vi "PicoScope5000aExampleRapidBlockBulkOverlapped.vi"() -> ()   [LabVIEW 2020]
uses:
  shared/Acquisition Settings.ctl
  shared/Buffer and Transfer Settings.ctl
  shared/nSegments.ctl
  shared/Segment Range.ctl
  PicoScope5000aLib/PicoScope5000aAnalogChannelSettings.ctl
  PicoScope5000aLib/PicoScope5000aDigitalChannelSettings.ctl
  shared/PicoBuffers.ctl
  <vilib>/Waveform/DWDTOps.llb/DWDT Analog to Digital.vi
panel:
  out "overflow":i16[](array[numeric]) format="%06b"
  in  "Port 0 Settings":T1={"Enabled"=FALSE, "Logic Level"=9830} {"Logic Level" items=["1.5V TTL"=9830, "2.5V CMOS"=16383]}
  in  "Channel A Settings":T2={"Enabled"=TRUE, "Coupling"=1, "Range"=6, "Analogue Offset"=0.0, "Bandwidth Limit"=0} {"Bandwidth Limit" items=["Full", "20MHz"]; "Range" items=["10 mV", "20 mV", "50 mV", "100 mV", "200 mV", "500 mV", "1 V", "2 V", "5 V", "10 V", "20 V"]; "Coupling" items=["AC", "DC"]}
  in  "Trigger Settings":T3={"Trigger Enabled"=FALSE, "Trigger Source"=enum."Channel A", "Trigger Threshold (volts)"=0.0, "Trigger Direction"=2, "Trigger Delay (samples)"=0, "Auto Trigger Time (ms)"=1000} {"Trigger Direction" items=["Rising"=2, "Falling"=3]}
  out "USB 3.0 device on non-USB 3.0 Port":bool
  out "USB Powered":bool=TRUE
  out "Device Info":T4={"Driver Version"="2.1.104.3324", "USB Version"="2.0", "Hardware"="1", "Variant"="5244A", "Batch and Serial"="CQ178/007", "Cal Date"="11Jun13", "Kernel Version"="1.0", "Digital HW Version"="1", "Analogue HW Version"="1", "MSO"=FALSE, "Number of channels"=2}
  out "Trigger Offsets":cluster{"Samples":u64, "Time (seconds)":sgl}[](array[cluster]) {"Time (seconds)" format="%#_5p"}
  in  "Stop Display":bool
  out "Capture Complete":bool
  in  "Run":bool
  in  "Display Buffer Index":i32
  in  "Segment Range":T5={"fromSegmentIndex"=0, "toSegmentIndex"=9} {"toSegmentIndex" format="%.4p"; "fromSegmentIndex" format="%.4p"}
  in  "nSegments":T6=10 format="%.4p"
  out "error out":errorcluster
  in  "Data file":path=path "PicoScope5000aExampleRapidBlock ChA Data"
  in  "Buffer and Transfer Settings":T7={"startIndex"=0, "Samples"=5000000, "Down Sample Ratio"=1, "Down-Sample Mode"=0} {"Down-Sample Mode" items=["RAW none"=2147483648, "None"=0, "Aggregate"=1, "Decimate"=2, "Average"=4]; "Down Sample Ratio" step=1; "Samples" format="%_6p"}
  in  "Acquisition Settings":T8={"preTriggerSamples"=0, "postTriggerSamples"=5000000, "timebase"=5} {"postTriggerSamples" format="%_6p"; "preTriggerSamples" format="%_6p"}
  out "Properties Panel":T9={"Sample Frequency"=41666668.0, "Sample Rate"=2.4000000209412065e-08, "Max Samples Available"=26843008, "Number of Samples"=0, "Total Capture Time (sec) "=0.0, "Max Total Capture Time Available (sec)"=0.6442322134971619} {"Max Total Capture Time Available (sec)" format="%.3p"; "Sample Frequency" format="%.6p"; "Sample Rate" format="%.3p"; "Max Samples Available" format="%_6p"; "Total Capture Time (sec)" format="%.3p"}
  out "Port 0":digitalwaveform(graph)={"t0"=timestamp(0 s since 1904-01-01), "dt"=8e-09, "Y"={"transitions"=[], "data"=[]}}
  in  "stop":bool
  out "Analog Channels":cluster{i32, sgl, "Data":dbl[]}[](graph)
  in  "Resolution":u32(ring) items=["8-bit"=0, "12-bit"=1, "14-bit"=2, "15-bit"=3, "16-bit"=4, "10-bit"=10]
  in  "Serial Number":string
  in  "Use Serial Number":bool
  in  "error in (no error)":errorcluster
  # "Number of\nSegments to Capture"
  # "Bit 0 = ChA"
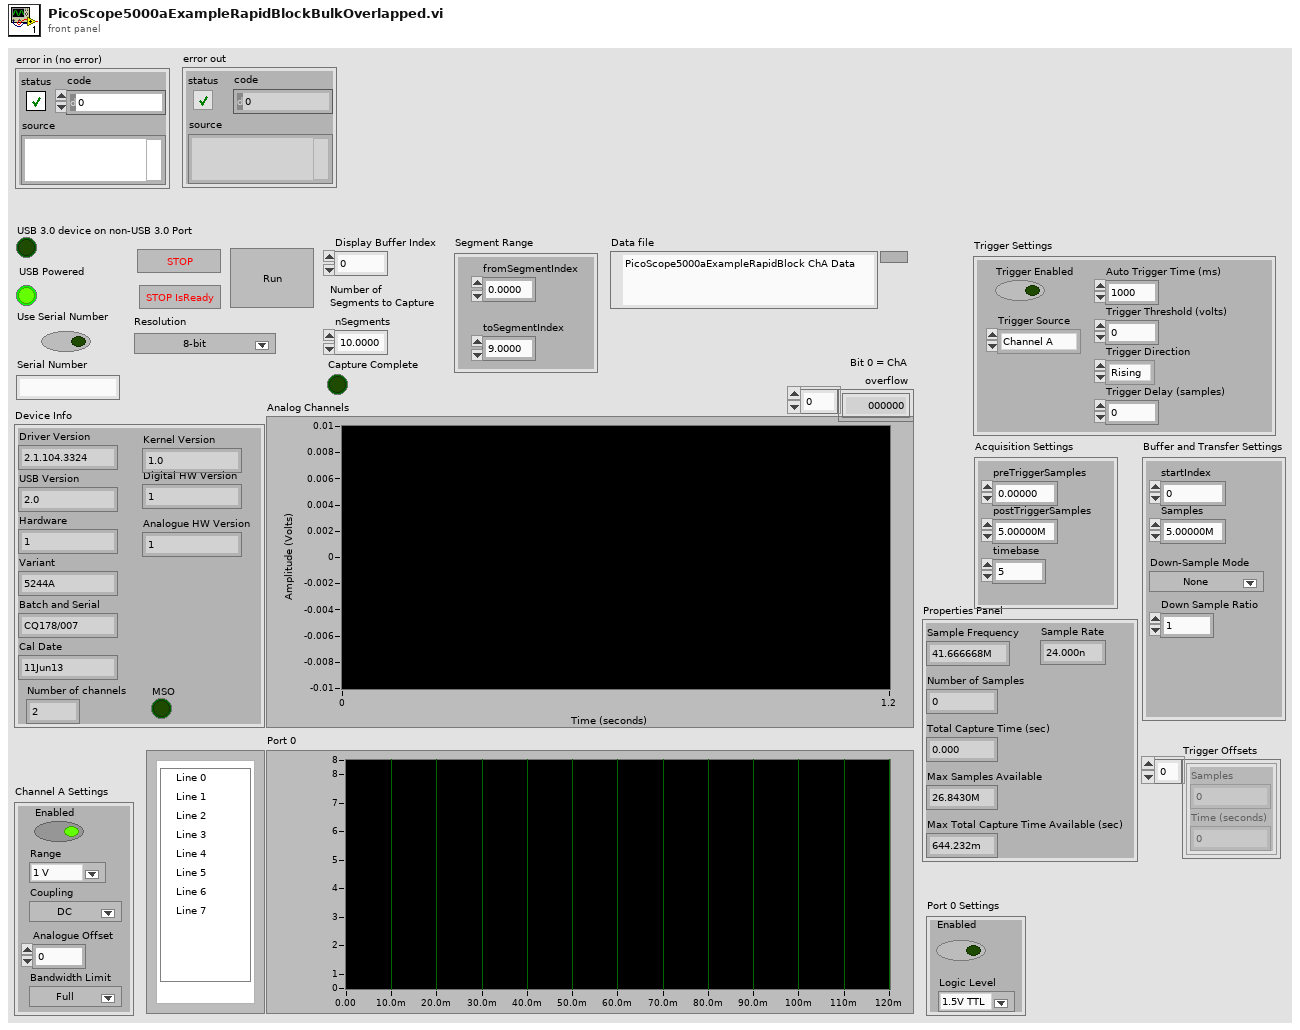
[diagram p1: front panel]
types:
  T1 = typedef "PicoScope5000aDigitalChannelSettings.ctl" = cluster{"Enabled":bool, "Logic Level":i16}
  T2 = typedef "PicoScope5000aAnalogChannelSettings.ctl" = cluster{"Enabled":bool, "Coupling":i16, "Range":u16, "Analogue Offset":sgl, "Bandwidth Limit":u32}
  T3 = cluster{"Trigger Enabled":bool, "Trigger Source":enum16{"Channel A", "Channel B", "Channel C", "Channel D", "Ext."}, "Trigger Threshold (volts)":dbl, "Trigger Direction":u16, "Trigger Delay (samples)":u32, "Auto Trigger Time (ms)":i16}
  T4 = cluster{"Driver Version":string, "USB Version":string, "Hardware":string, "Variant":string, "Batch and Serial":string, "Cal Date":string, "Kernel Version":string, "Digital HW Version":string, "Analogue HW Version":string, "MSO":bool, "Number of channels":i16}
  T5 = typedef "Segment Range.ctl" = cluster{"fromSegmentIndex":u64, "toSegmentIndex":u64}
  T6 = typedef "nSegments.ctl" = u64
  T7 = typedef "Buffer and Transfer Settings.ctl" = cluster{"startIndex":u64, "Samples":u64, "Down Sample Ratio":u64, "Down-Sample Mode":u32}
  T8 = typedef "Acquisition Settings.ctl" = cluster{"preTriggerSamples":u64, "postTriggerSamples":u64, "timebase":u32}
  T9 = cluster{"Sample Frequency":dbl, "Sample Rate":dbl, "Max Samples Available":u64, "Number of Samples":u64, "Total Capture Time (sec) ":dbl, "Max Total Capture Time Available (sec)":dbl}
  T10 = enum16{"open", "open or create", "create or replace", "create", "open (read-only)"}
  T11 = typedef "PicoBuffers.ctl" = cluster{"Max Buffer Pointers":u64[][][], "Min Buffer Pointers":u64[][][], "StreamingDataInfo":cluster{"Channel":u32, "Down-Sample Mode":u32, "PICO_DATA_TYPE":enum32{"PICO_INT8_T", "PICO_INT16_T", "PICO_INT32_T", "PICO_UINT32_T", "PICO_INT64_T", ""}, "Samples":i32, "bufferIndex":u64, "startIndex":i32, "overflow":i16}[][]}
  T12 = cluster{"Sample Frequency":sgl, "Sample Rate":sgl, "Max Samples Available":i32, "Number of Samples":u32, "Total Capture Time (sec) ":sgl, "Max Total Capture Time Available (sec)":sgl}
  T13 = cluster{"Channel A Buffer":i16[], "Channel B Buffer":i16[], "Channel C Buffer":i16[], "Channel D Buffer":i16[], "Channel E Buffer":i16[], "Channel F Buffer":i16[], "Channel G Buffer":i16[], "Channel H Buffer":i16[], "Port 0 Buffer":i16[], "Port 1 Buffer":i16[]}[]
  T14 = cluster{"Channel A Buffer":i16[], "Channel B Buffer":i16[], "Channel C Buffer":i16[], "Channel D Buffer":i16[], "Channel E Buffer":i16[], "Channel F Buffer":i16[], "Channel G Buffer":i16[], "Channel H Buffer":i16[], "Port 0 Buffer":i16[], "Port 1 Buffer":i16[]}
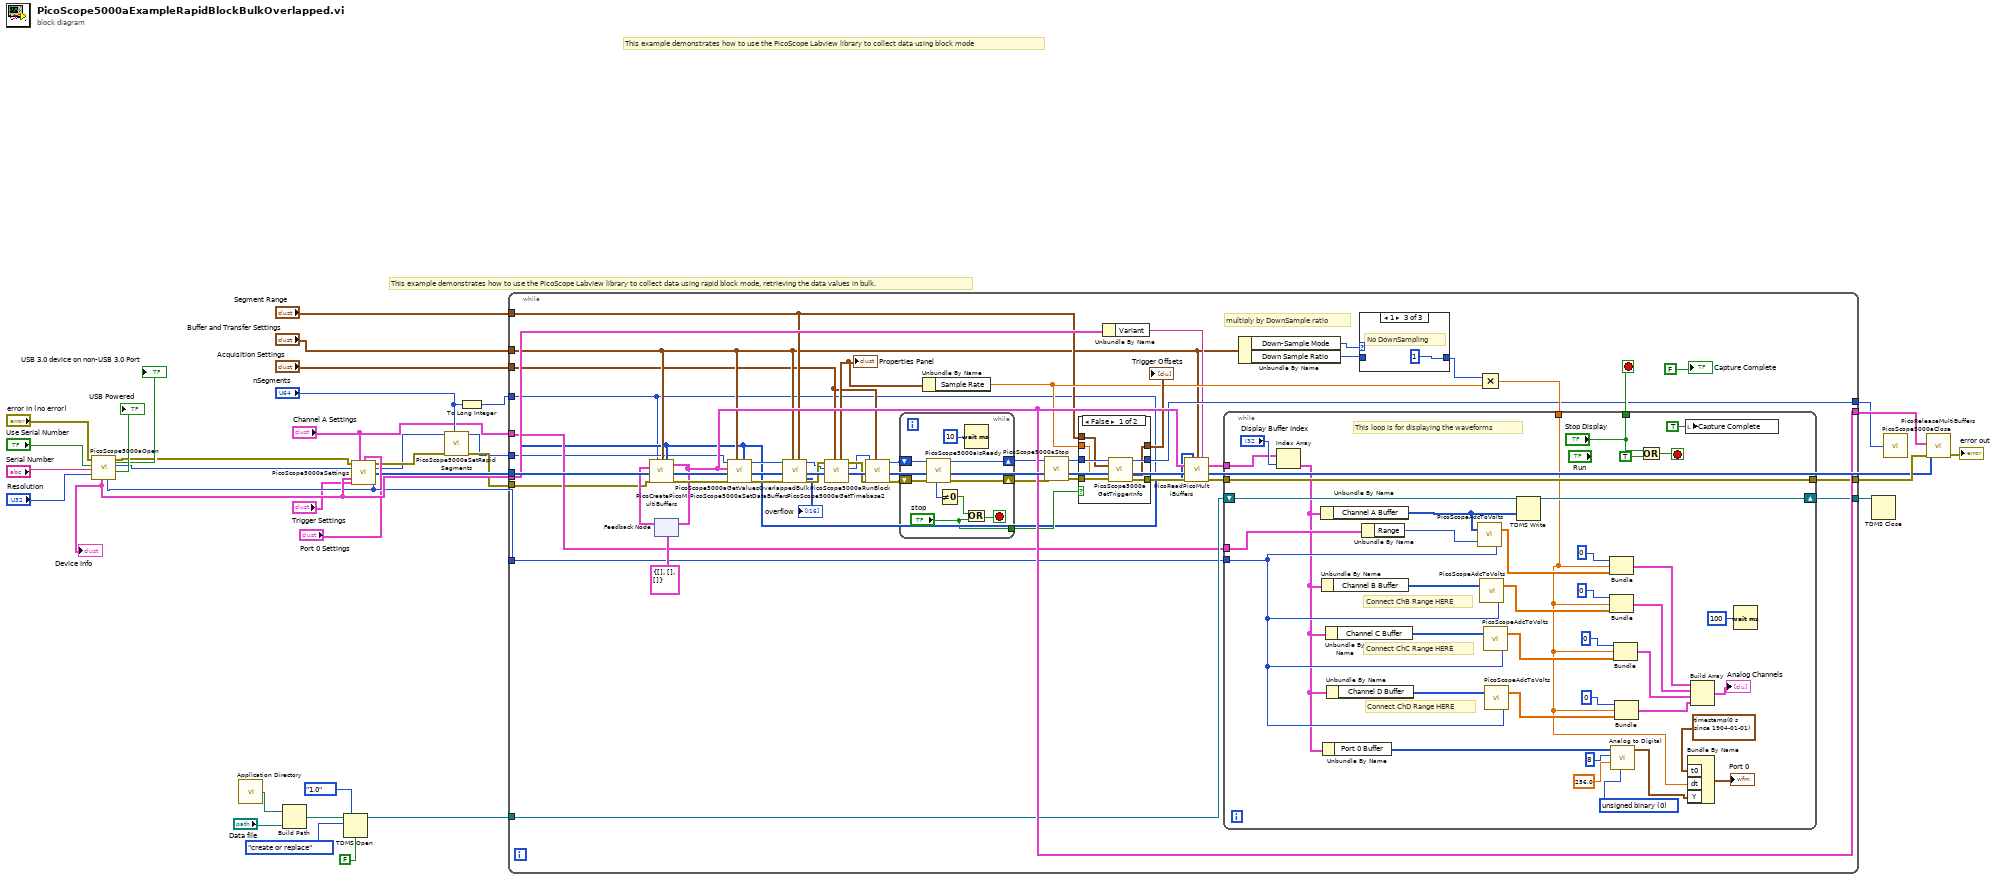
[diagram p0: block diagram]
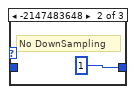
[diagram p4: hidden frame]
diagram:
  # "This example demonstrates how to use the PicoScope Labview library to collect data using rapid block mode, retrieving the data values in bulk."
  # "This example demonstrates how to use the PicoScope Labview library to collect data using block mode"
  n1 = call "PicoScope5000aOpen.vi"("Serial Number"="Serial Number", "Resolution"="Resolution", "Use Serial Number"="Use Serial Number", "error in (no error)"="error in (no error)") -> ("USB Powered"=→"USB Powered":bool, "handle"=w8:i16, "error out"=w10:errorcluster, "Max ADC value"=w19:i16, "USB 3.0 device on non-USB 3.0 Port"=→"USB 3.0 device on non-USB 3.0 Port":bool, "Device Info"=w20:T4)  [unwired: 2 in]
  "Device Info" <- w20
  n2 = call <vilib>:"Application Directory.vi"() -> ("Application Directory"=w28:path)
  n3 = Build Path(base path=w28, name or relative path="Data file") -> (appended path=w29:path)
  n4 = TDMS Open(6:FALSE ("disable buffering? (T)"), 7:enum16{"1.0", "2.0"}."1.0" ("file format version (2.0)"), 10:T10."create or replace" ("operation (0:open)"), 11:w29) -> (3:w26:refnum<k34>)  [unwired: 3 in, 1 out]
  n5 = call "PicoScope5000aSettings.vi"("error in"=w10, "Channel A Settings"="Channel A Settings", "Port 0 Settings"="Port 0 Settings", "handle in"=w8, "Device Info"=w20, "Trigger Settings"="Trigger Settings", "Max ADC value"=w19) -> ("error out"=w5:errorcluster, "handle out"=w4:i16, "enabled array"=w6:i16[])  [unwired: 6 in]
  n6 = call "PicoScope5000aSetRapidSegments.vi"("nSegments"="nSegments", "error in (no error)"=w5, "handle in"=w4) -> ("error out"=w3:errorcluster, "handle out"=w2:i16)  [unwired: 6 in, 1 out]
  n7 = To Long Integer(number="nSegments") -> (32bit integer=w1:i32)
  n8 = while {
    tunnel: w19 -> [w48]
    tunnel: [w60] -> w34
    tunnel: [w77] -> w35
    tunnel: [w76] -> w27
    tunnel: w26 -> [w75]
    tunnel: w20 -> [w44]
    tunnel: [w50] -> w16
    tunnel: "Segment Range" -> [w43]
    tunnel: "Buffer and Transfer Settings" -> [w42]
    tunnel: "Acquisition Settings" -> [w41]
    tunnel: "Channel A Settings" -> [w40]
    tunnel: w6 -> [w39]
    tunnel: w3 -> [w38]
    tunnel: w2 -> [w37]
    tunnel: w1 -> [w36]
    stop <- w63 stop-if-true
    # "multiply by DownSample ratio"
    n9 = feedback #1(T11 {"Max Buffer Pointers"=[], "Min Buffer Pointers"=[], "StreamingDataInfo"=[]} ("Data Pointers")) -> (w79:T11)
    n10 = call "PicoCreatePicoMultiBuffers.vi"("Number of Buffers"=w36, "Buffer and Transfer Settings"=w42, "enabled array"=w39, "Data Pointers In"=w79, "error in (no error)"=w38) -> ("Data Pointers"=w77:T11, "error out"=w78:errorcluster)  [unwired: 9 in]
    n11 = feedback-in #1(w77) -> ()
    n12 = call "PicoScope5000aSetDataBuffers.vi"("enabled array"=w39, "Buffer and Transfer Settings"=w42, "error in (no error)"=w78, "Data Pointers In"=w77, "handle in"=w37) -> ("error out"=w74:errorcluster, "handle out"=w73:i16)  [unwired: 5 in]
    n13 = call "PicoScope5000aGetValuesOverlappedBulk.vi"("Segment Range"=w43, "Buffer and Transfer Settings"=w42, "error in (no error)"=w74, "handle in"=w73) -> ("error out"=w54:errorcluster, "handle out"=w53:i16, "overflow"=→"overflow":i16[])  [unwired: 4 in, 1 out]
    n14 = call "PicoScope5000aGetTimebase2.vi"("Acquisition Settings"=w41, "handle in"=w53, "error in (no error)"=w54) -> ("handle out"=w51:i16, "error out"=w52:errorcluster, "Properties Panel"=w69:T12)  [unwired: 6 in]
    "Properties Panel" <- w69
    n15 = call "PicoScope5000aRunBlock.vi"("Acquisition Settings"=w41, "error in (no error)"=w52, "handle in"=w51) -> ("error out"=w66:errorcluster, "handle out"=w65:i16)  [unwired: 5 in, 2 out]
    n16 = while {
      shift-right: [w136] -> w58
      shift-left: w66 -> [w137]
      shift-right: [w135] -> w55
      shift-left: w65 -> [w134]
      tunnel: ["stop"] -> w47
      stop <- w130 stop-if-true
      n17 = call "PicoScope5000aIsReady.vi"("error in (no error)"=w137, "handle in"=w134) -> ("error out"=w136:errorcluster, "handle out"=w135:i16, "ready"=w132:i16)  [unwired: 7 in]
      n18 = Not Equal To 0?(x=w132) -> (x != 0?=w131:bool)
      n19 = Wait (ms)(milliseconds to wait=u32 10) -> ()  [unwired: 1 out]
      n20 = Or(x=w131, y="stop") -> (x .or. y?=w130:bool)
    }
    n21 = Unbundle By Name(w69) -> ("Sample Rate"=w46:sgl)
    n22 = call "PicoScope5000aStop.vi"("error in (no error)"=w58, "handle in"=w55) -> ("error out"=w57:errorcluster, "handle out"=w56:i16)  [unwired: 8 in]
    n23 = case shown="False" w47 {
      tunnel: [w87 w88] -> w61
      tunnel: [w86 w89] -> w60
      tunnel: [w85 _] -> w59
      tunnel: w57 -> [w84 w88]
      tunnel: w56 -> [w83 w89]
      tunnel: w43 -> [w82 _]
      tunnel: w46 -> [w81 _]
      frame False {
        n24 = call "PicoScope5000aGetTriggerInfo.vi"("handle in"=w83, "Rapid Block Acquisition Settings"=w82, "Sample Rate"=w81, "error in"=w84) -> ("handle out"=w86:i16, "Trigger Offsets"=w85:cluster{u64, sgl}[], "error out"=w87:errorcluster)  [unwired: 8 in, 1 out]
      }
      frame True {
      }
    }
    "Trigger Offsets" <- w59
    n25 = Unbundle By Name(w44) -> ("Variant"=w45:string)
    n26 = call "PicoReadPicoMultiBuffers.vi"("enabled array"=w39, "Buffer and Transfer Settings"=w42, "Variant"=w45, "Data Pointers"=w77, "No of Buffers"=w36, "error in (no error)"=w61) -> ("MultiBuffers (Max or non-aggregated)"=w72:T13, "error out"=w64:errorcluster)  [unwired: 7 in, 1 out]
    n27 = Unbundle By Name(w42) -> ("Down-Sample Mode"=w70:u32, "Down Sample Ratio"=w71:u64)
    n28 = case shown="1" w70 {
      tunnel: [w138 u64 1 ("Down Sample Ratio") u64 1 ("Down Sample Ratio")] -> w67
      tunnel: w71 -> [w138 _ _]
      frame Default {
      }
      frame -2147483648 {
        # "No DownSampling"
      }
      frame 1 {
        # "No DownSampling"
      }
    }
    n29 = Multiply(x=w67, y=w46) -> (x*y=w68:sgl)
    n30 = while {
      tunnel: w48 -> [w92]
      tunnel: w40 -> [w128]
      tunnel: w72 -> [w102]
      tunnel: w68 -> [w94]
      shift-right: [w127] -> w76
      shift-left: w75 -> [w126]
      tunnel: [w107] -> w50
      tunnel: w64 -> [w107]
      tunnel: ["Stop Display"] -> w63
      stop <- w105 stop-if-true
      w116 = u16 0 items=["unsigned binary", "offset binary", "2's complement"] ("data format (offset binary)")
      # "This loop is for displaying the waveforms"
      # "Connect ChB Range HERE"
      # "Connect ChD Range HERE"
      # "Connect ChC Range HERE"
      n31 = Index Array(array=w102, index="Display Buffer Index") -> (element=w91:T14)
      n32 = Unbundle By Name(w91) -> ("Channel A Buffer"=w109:i16[])
      n33 = Unbundle By Name(w91) -> ("Channel B Buffer"=w122:i16[])
      n34 = Unbundle By Name(w91) -> ("Port 0 Buffer"=w114:i16[])
      n35 = Unbundle By Name(w91) -> ("Channel C Buffer"=w100:i16[])
      n36 = Unbundle By Name(w91) -> ("Channel D Buffer"=w96:i16[])
      n37 = Unbundle By Name(w128) -> ("Range"=w124:u16)
      n38 = call "PicoScopeAdcToVolts.vi"("Max_adc"=w92, "Range Index"=w124, "Data"=w109) -> ("Data"=w110:dbl[])
      n39 = call "PicoScopeAdcToVolts.vi"("Max_adc"=w92, "Data"=w122) -> ("Data"=w121:dbl[])  [unwired: 1 in]
      n40 = call "PicoScopeAdcToVolts.vi"("Max_adc"=w92, "Data"=w100) -> ("Data"=w99:dbl[])  [unwired: 1 in]
      n41 = call "PicoScopeAdcToVolts.vi"("Max_adc"=w92, "Data"=w96) -> ("Data"=w95:dbl[])  [unwired: 1 in]
      n42 = TDMS Write(0:w126, 9:w109) -> (4:w127:refnum<k34>)  [unwired: 4 in, 3 out]
      n43 = Bundle(0, w94, "Data"=w110) -> (w120:cluster{i32, sgl, "Data":dbl[]})  [unwired: 1 in]
      n44 = Bundle(0, w94, "Data"=w121) -> (w119:cluster{i32, sgl, "Data":dbl[]})  [unwired: 1 in]
      n45 = call-poly <vilib>:"Analog to Digital.vi"("data format (offset binary)"=w116, "full-scale range (pk-pk)"=256.0, "resolution (16 bit)"=8, "analog waveform"=w114) -> ("digital waveform"=w111:digitalwaveform)  [unwired: 4 in, 3 out]
      n46 = Bundle(0, w94, "Data"=w99) -> (w98:cluster{i32, sgl, "Data":dbl[]})  [unwired: 1 in]
      n47 = Bundle(0, w94, "Data"=w95) -> (w93:cluster{i32, sgl, "Data":dbl[]})  [unwired: 1 in]
      n48 = Or(x="Stop Display", y=TRUE) -> (x .or. y?=w105:bool)
      n49 = local write "Capture Complete"(TRUE ("Capture Complete")) -> ()
      n50 = Bundle By Name("t0"=timestamp(0 s since 1904-01-01), "dt"=w94, "Y"=w111) -> (→"Port 0":digitalwaveform)  [unwired: 1 in]
      n51 = Build Array(w120, w119, w98, w93) -> (→"Analog Channels":cluster{i32, sgl, "Data":dbl[]}[])
      n52 = Wait (ms)(milliseconds to wait=u32 100) -> ()  [unwired: 1 out]
    }
    "Capture Complete" <- FALSE ("Capture Complete")
  }
  n53 = TDMS Close(11:w27) -> ()  [unwired: 1 in, 2 out]
  n54 = call "PicoScope5000aClose.vi"("handle"=w34) -> ()
  n55 = call "PicoReleaseMultiBuffers.vi"("error in (no error)"=w16, "Enabled array"=w6, "Data Pointers"=w35) -> ("error out"=→"error out":errorcluster)  [unwired: 8 in]
